vi "BRig_Host_dataRunState_idx_trig_l1.vi"() -> (2 "output_idx_trig_l1":i32)   [LabVIEW 2014]
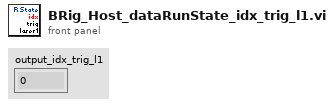
[diagram p1: front panel]
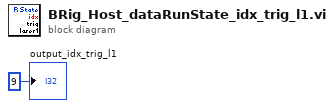
[diagram p0: block diagram]
diagram:
  "output_idx_trig_l1" <- 9 ("output_idx_dataTS")
